vi "Sonar.vi"() -> ()   [LabVIEW 2011]
uses:
  <vilib>/Rock Robotics/SystemInterfaces/Typedef/FPGA_TypedefAnalogModule.ctl
panel:
  out "distance":dbl(slide)=125.0 scale=0.0..250.0 scale format="%3d"
  # "feet"
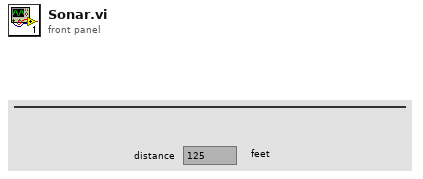
[diagram p1: front panel]
types:
  T1 = typedef "FPGA_TypedefAnalogModule.ctl" = enum16{"Analog Module 1", "Analog Module 2"}
  T2 = typedef "WPI_AnalogChannelDevRef.ctl" = cluster{"DevStatus":errorcluster, "Analog Module":T1, "Analog Channel":T3}
  T3 = typedef "FPGA_AIChannel.ctl" = enum8{"AI 1", "AI 2", "AI 3", "AI 4", "AI 5", "AI 6", "AI 7", "AI 8", "Invalid"}
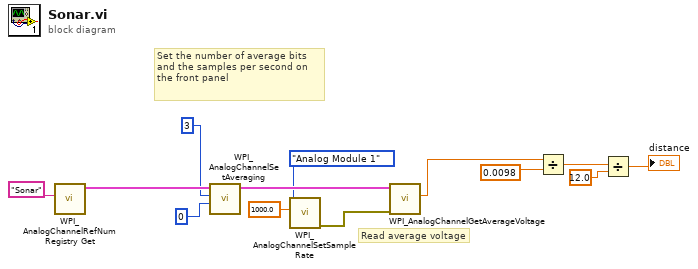
[diagram p0: block diagram]
diagram:
  # "Read average voltage"
  # "Set the number of average bits and the samples per second on the front panel"
  n1 = call <vilib>:"WPI_AnalogChannelRefNum Registry Get.vi"("refnum name"="Sonar") -> ("AIDeviceRef"=w5:T2)  [unwired: 9 in, 1 out]
  n2 = call <vilib>:"WPI_AnalogChannelSetAveraging.vi"("OversampleBits"=u8 0, "AverageBits"=u8 3, "AIDeviceRef"=w5) -> ("AIDeviceRef"=w11:T2)  [unwired: 1 in, 7 out]
  n3 = call <vilib>:"WPI_AnalogChannelSetSampleRate.vi"("Samples Per Second"=1000.0, "Analog Module (Module 1)"=FPGA_TypedefAnalogModule."Analog Module 1") -> ("error out"=w10:errorcluster)  [unwired: 2 in, 7 out]
  n4 = call <vilib>:"WPI_AnalogChannelGetAverageVoltage.vi"("error in (no error)"=w10, "AIDeviceRef"=w11) -> ("Voltage"=w1:dbl)  [unwired: 9 out]
  n5 = Divide(x=w1, y=0.0098) -> (x/y=w8:dbl)
  n6 = Divide(x=w8, y=12.0) -> (x/y=→"distance":dbl)
